vi "UnregisterMat_2DArray-EXT.vi"(6 "AdressOrData":ext[][](array[numeric]), 8 "error in":errorcluster, 11 "Image":u8) -> (0 "error out":errorcluster, 3 "Datatype":ext[][](array[numeric]))   [LabVIEW 2020, in "OpenLvVision_OpenCv.lvlib"]
doc: "Register mat for dll.\nNo malleable to breake vi inlining!"
uses:
  OpenLvVision_OpenCv.lvlib
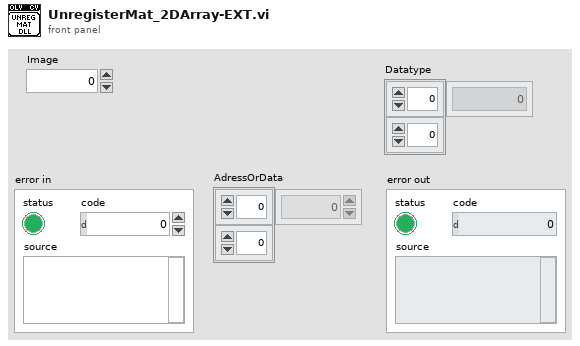
[diagram p1: front panel]
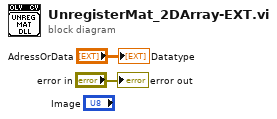
[diagram p0: block diagram]
diagram:
  "error out" <- "error in"
  "Datatype" <- "AdressOrData"
